vi "Mark Trace.vi"(8 "error in (no error)":errorcluster, 10 "Trace Marker":T1, 11 "SequenceViewPanel in":refnum<class "SequenceViewPanel.lvclass">) -> (0 "error out":errorcluster, 3 "SequenceViewPanel out":refnum<class "SequenceViewPanel.lvclass">)   [LabVIEW 2020, in "TSnax UI.lvlib" / "SequenceViewPanel.lvclass"]
uses:
  SequenceViewPanel.lvclass
  Trace Marker.ctl
  TSnax/SequenceFile/SequenceFile.lvclass
  Mark Trace Data.ctl
  SequenceViewPanel.lvclass/SequenceViewPanel.ctl
  5042c8d5-d480-43a7-b921-b0c156911035.vi
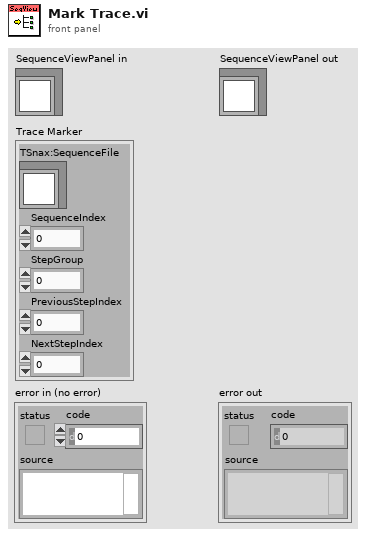
[diagram p1: front panel]
types:
  T1 = typedef "TSnax UI.lvlib/SequenceViewPanel.lvclass/Trace Marker.ctl" = cluster{"TSnax:SequenceFile":refnum<class "SequenceFile.lvclass">, "SequenceIndex":i32, "StepGroup":i32, "PreviousStepIndex":i32, "NextStepIndex":i32}
  T2 = typedef "TSnax UI.lvlib/SequenceViewPanel.lvclass/Mark Trace Data.ctl" = cluster{"Trace Marker":T1}
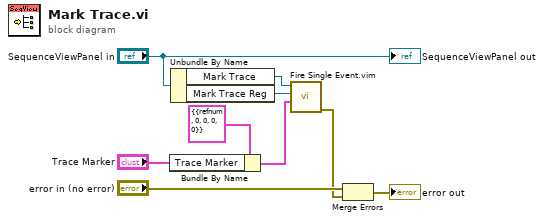
[diagram p0: block diagram]
diagram:
  n1 = Bundle By Name(cluster=T2 {"Trace Marker"={"TSnax:SequenceFile"=refnum, "SequenceIndex"=0, "StepGroup"=0, "PreviousStepIndex"=0, "NextStepIndex"=0}} ("Mark Trace Data"), "Trace Marker"="Trace Marker") -> (w1:T2)
  n2 = Unbundle By Name("SequenceViewPanel in") -> ("Mark Trace"=w5:refnum<user-event>, "Mark Trace Reg"=w4:refnum<event-registration>)
  n3 = call "Fire Single Event.vim"("Data"=w1, "Event Reg"=w4, "Event"=w5) -> ("error out"=w6:errorcluster)  [unwired: 8 in]
  n4 = Merge Errors("error in (no error)", w6) -> (→"error out":errorcluster)
  "SequenceViewPanel out" <- "SequenceViewPanel in"
